vi "Punto 4.vi"() -> ()   [LabVIEW 2020]
panel:
  out "Unpair numbers":dbl
  out "Pair numbers":dbl
  in  "Stop buttom":bool
  out "Final array":string[](array[string])
  in  "Operate":bool
  in  "Original arrray":dbl[](array[numeric])
  in  "Array 3":string[](array[string])
  # "This program was created by Juan Bermúdez from the Army Aviation School\nat the Aircraft Engineering of the assignature of Programation II"
  # "How to use the software?:\n1- First, write the numbers.\n2- Second, push the buttom called = ''Operate''.\n3- Third, if you want to stop the software, push the buttom called = ''Stop buttom''.\n Enjoy the software :)"
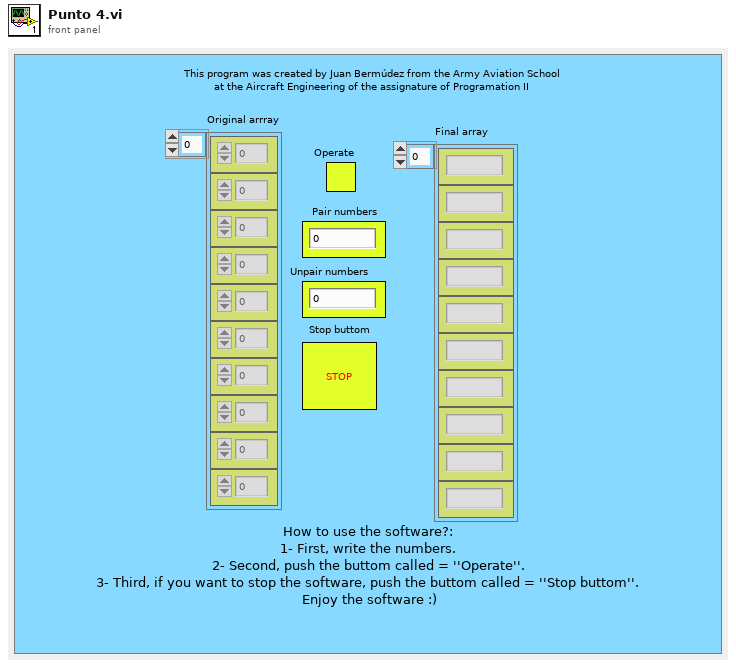
[diagram p1: front panel]
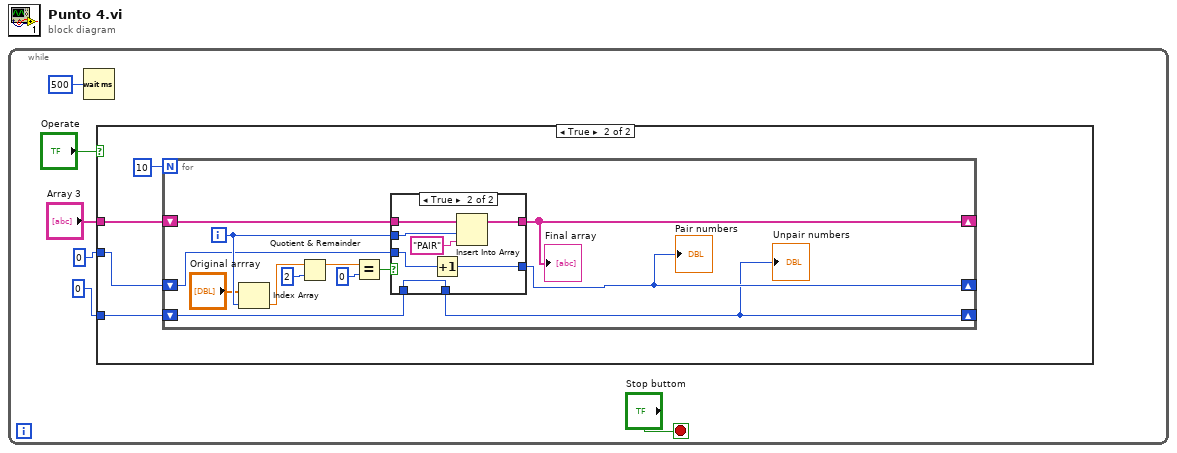
[diagram p0: block diagram]
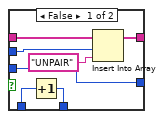
[diagram p3: hidden frame]
diagram:
  n1 = while {
    stop <- "Stop buttom" stop-if-true
    n2 = Wait (ms)(milliseconds to wait=u32 500) -> ()  [unwired: 1 out]
    n3 = case shown="True" "Operate" {
      tunnel: "Array 3" -> [_ w9]
      tunnel: 0 -> [_ w8]
      tunnel: 0 -> [_ w7]
      frame False {
      }
      frame True {
        n4 = for {
          N: 10 -> [_]
          shift-right: [w16] -> _
          shift-left: w9 -> [w15]
          shift-right: [w12] -> _
          shift-left: w8 -> [w14]
          shift-right: [w11] -> _
          shift-left: w7 -> [w13]
          i -> [w19]
          n5 = Index Array(array="Original arrray", index=w19) -> (element=w23:dbl)
          n6 = Quotient & Remainder(x=w23, y=2) -> (x-y*floor(x/y)=w17:dbl)  [unwired: 1 out]
          n7 = Equal?(x=w17, y=0) -> (x = y?=w20:bool)
          n8 = case shown="True" w20 {
            tunnel: w19 -> [w27 w37]
            tunnel: w15 -> [w28 w36]
            tunnel: [w29 w34] -> w16
            tunnel: w14 -> [w24 w33]
            tunnel: [w24 w32] -> w12
            tunnel: w13 -> [w26 w31]
            tunnel: [w25 w31] -> w11
            frame False {
              n9 = Increment(x=w26) -> (x+1=w25:i32)
              n10 = Insert Into Array(array=w28, index=w27, new element="UNPAIR") -> (w29:string[])
            }
            frame True {
              n11 = Increment(x=w33) -> (x+1=w32:i32)
              n12 = Insert Into Array(array=w36, index=w37, new element="PAIR") -> (w34:string[])
            }
          }
          "Final array" <- w16
          "Pair numbers" <- w12
          "Unpair numbers" <- w11
        }
      }
    }
  }
